vi "Test.ml.vi"(0 "n":i32, 1 "mlp":u64, 2 "MathLink Dll":path) -> ()   [LabVIEW 2014]
uses:
  ml64i4.dll
panel:
  out "Array":variant[](array[variant])
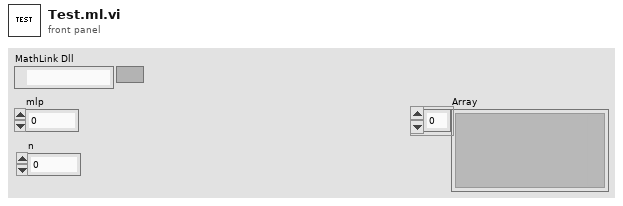
[diagram p1: front panel]
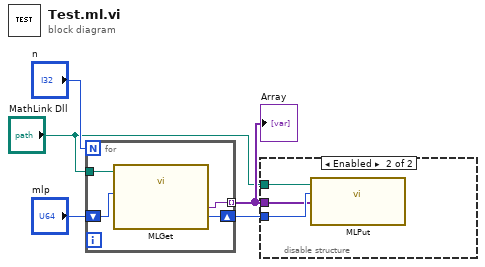
[diagram p0: block diagram]
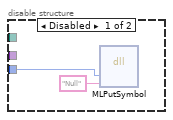
[diagram p2: hidden frame]
diagram:
  n1 = for {
    N: "n" -> [_]
    shift-right: [w8] -> w4
    shift-left: "mlp" -> [w9]
    tunnel: [w7] -> w3 mode=indexing
    tunnel: "MathLink Dll" -> [w6]
    n2 = call "MLGet.vi"("mlp in"=w9, "MathLink Dll"=w6) -> ("Variant"=w7:variant, "mlp out"=w8:u64)  [unwired: 1 in, 4 out]
  }
  "Array" <- w3
  n3 = disable-structure shown="Enabled" {
    disable-tunnel: w4 -> [w10 w14]
    disable-tunnel: w3 -> [_ w13]
    disable-tunnel: "MathLink Dll" -> [_ w12]
    frame Disabled {
      n4 = dll-call lib="ml64i4.dll" fn="MLPutSymbol"("mlp"=w10, "s"="Null") -> ()  [unwired: 6 in, 2 out]
    }
    frame Enabled {
      n5 = call "MLPut.vi"("Variant"=w13, "mlp in"=w14, "MathLink Dll"=w12) -> ()  [unwired: 1 in, 1 out]
    }
  }
